vi "Get TransferMode.vi"(8 "error in (no error)":errorcluster, 11 "FileTransferOptions in":refnum<class "FileTransferOptions.lvclass">) -> (0 "error out":errorcluster, 2 "TransferMode":T1, 3 "FileTransferOptions out":refnum<class "FileTransferOptions.lvclass">)   [LabVIEW 2015, in "WinSCP.lvlib" / "FileTransferOptions.lvclass"]
uses:
  FileTransferOptions.lvclass
  TransferMode.ctl
  FileTransferOptions.lvclass/FileTransferOptions.ctl
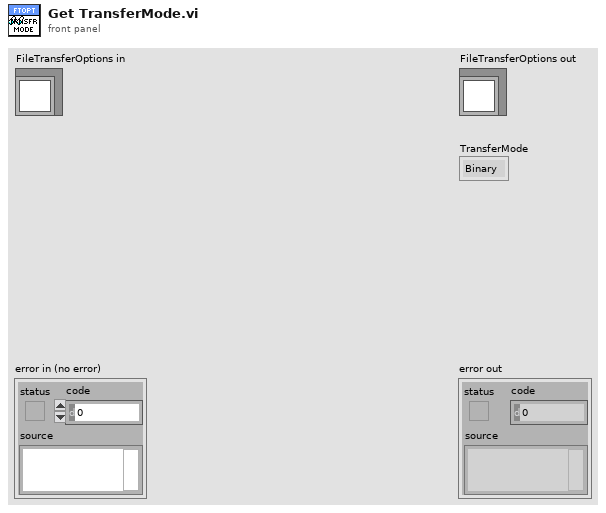
[diagram p1: front panel]
types:
  T1 = typedef "WinSCP.lvlib/FileTransferOptions.lvclass/TransferMode.ctl" = enum16{"Binary", "Ascii", "Auto"}
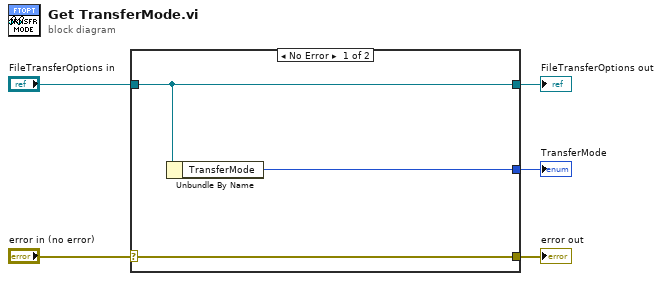
[diagram p0: block diagram]
diagram:
  n1 = case shown="No Error" "error in (no error)" {
    selector: "error in (no error)" -> [w8 w9]
    tunnel: [w8 w9] -> w4
    tunnel: [w7 w10] -> w2
    tunnel: "FileTransferOptions in" -> [w7 w10]
    tunnel: [w6 _] -> w1
    frame No Error {
      n2 = Unbundle By Name(w7) -> ("TransferMode"=w6:T1)
    }
    frame Error {
    }
  }
  "error out" <- w4
  "FileTransferOptions out" <- w2
  "TransferMode" <- w1
